vi "calcVectorField.vi"(7 "m":u32, 8 "error (in)":errorcluster, 10 "Boundary Points (1D)":cluster{"x":dbl, "y":dbl}[](array[cluster]), 11 "Interior Points (1D)":cluster{"x":dbl, "y":dbl}[](array[cluster])) -> (0 "error (out)":errorcluster, 1 "divergence(Fx, Fy)":dbl[][](array[numeric]), 2 "Y Vector Component":dbl[][](array[numeric]), 3 "X Vector Component":dbl[][](array[numeric]), 4 "curl(Fx, Fy)":dbl[][](array[numeric]))   [LabVIEW 2015]
uses:
  <vilib>/Analysis/baseanly.llb/Unit Vector (DBL).vi
  <vilib>/imath/engines/lvmath2/RunTimeEngine/Managers/WorkSpace/UID Generator.vi
  <vilib>/imath/engines/lvmath2/RunTimeEngine/BuiltInFunctions/divergence/NIMS_divergence(M,M).vi
  <vilib>/imath/engines/lvmath2/RunTimeEngine/RunTimeType/NIMS_RunTimeType_From StrictType (excl LVString).vi
  <instcachedir>/0/NIMS_RunTimeType_From StrictType (excl LVString)_EB1C38A9BC5048DA9ABDA8F781E54D21.lvgen/NIMS_RunTimeType_From StrictType (excl LVString)_EB1C38A9BC5048DA9ABDA8F781E54D21_000.vi
  <vilib>/imath/engines/lvmath2/RunTimeEngine/ErrorHandling/NIMS_Error From Error Code.vi
  <vilib>/imath/engines/lvmath2/RunTimeEngine/LocalVariableDefStatement/MC_LocalVariableDefStatement_Display.vi
  <vilib>/imath/engines/lvmath2/RunTimeEngine/BuiltInFunctions/curl/NIMS_[2o]_curl(M,M).vi
  <vilib>/imath/engines/lvmath2/RunTimeEngine/Managers/SymbolTable/Clear UID.vi
  <vilib>/imath/engines/lvmath2/RunTimeEngine/NodeEndStatement/NIMS_NodeEndStatement_Output.vi
  <instcachedir>/0/NIMS_NodeEndStatement_Output_53EC0D466D134D7ABD903AC30B43404B.lvgen/NIMS_NodeEndStatement_Output_53EC0D466D134D7ABD903AC30B43404B_002.vi
  <vilib>/imath/engines/lvmath2/RunTimeEngine/ErrorHandling/NIMS_Finalize Error.vi
  <vilib>/express/express arith-compare/Formula/XNode/ExpressFormulaBlockNode.xnode
  <vilib>/Analysis/NI_AALBase.lvlib
  <vilib>/imath/engines/lvmath2/RunTimeEngine/Managers/SymbolTable/NIMS_WorkSpace.lvlib
panel:
  out "-m":dbl
  out "m+2":dbl
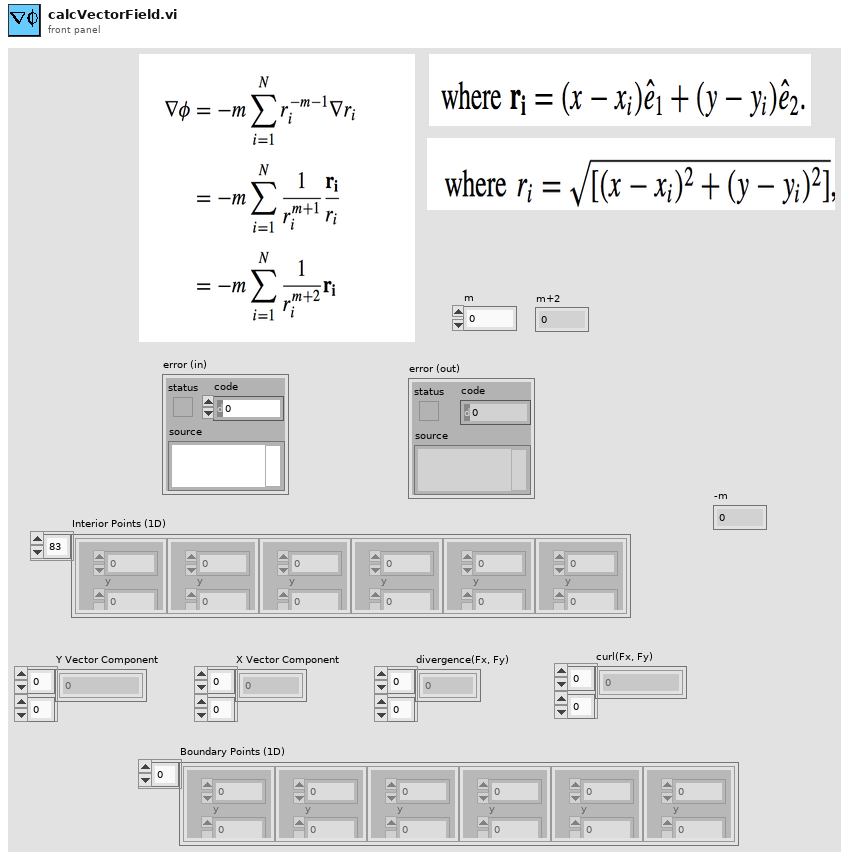
[diagram p1: front panel]
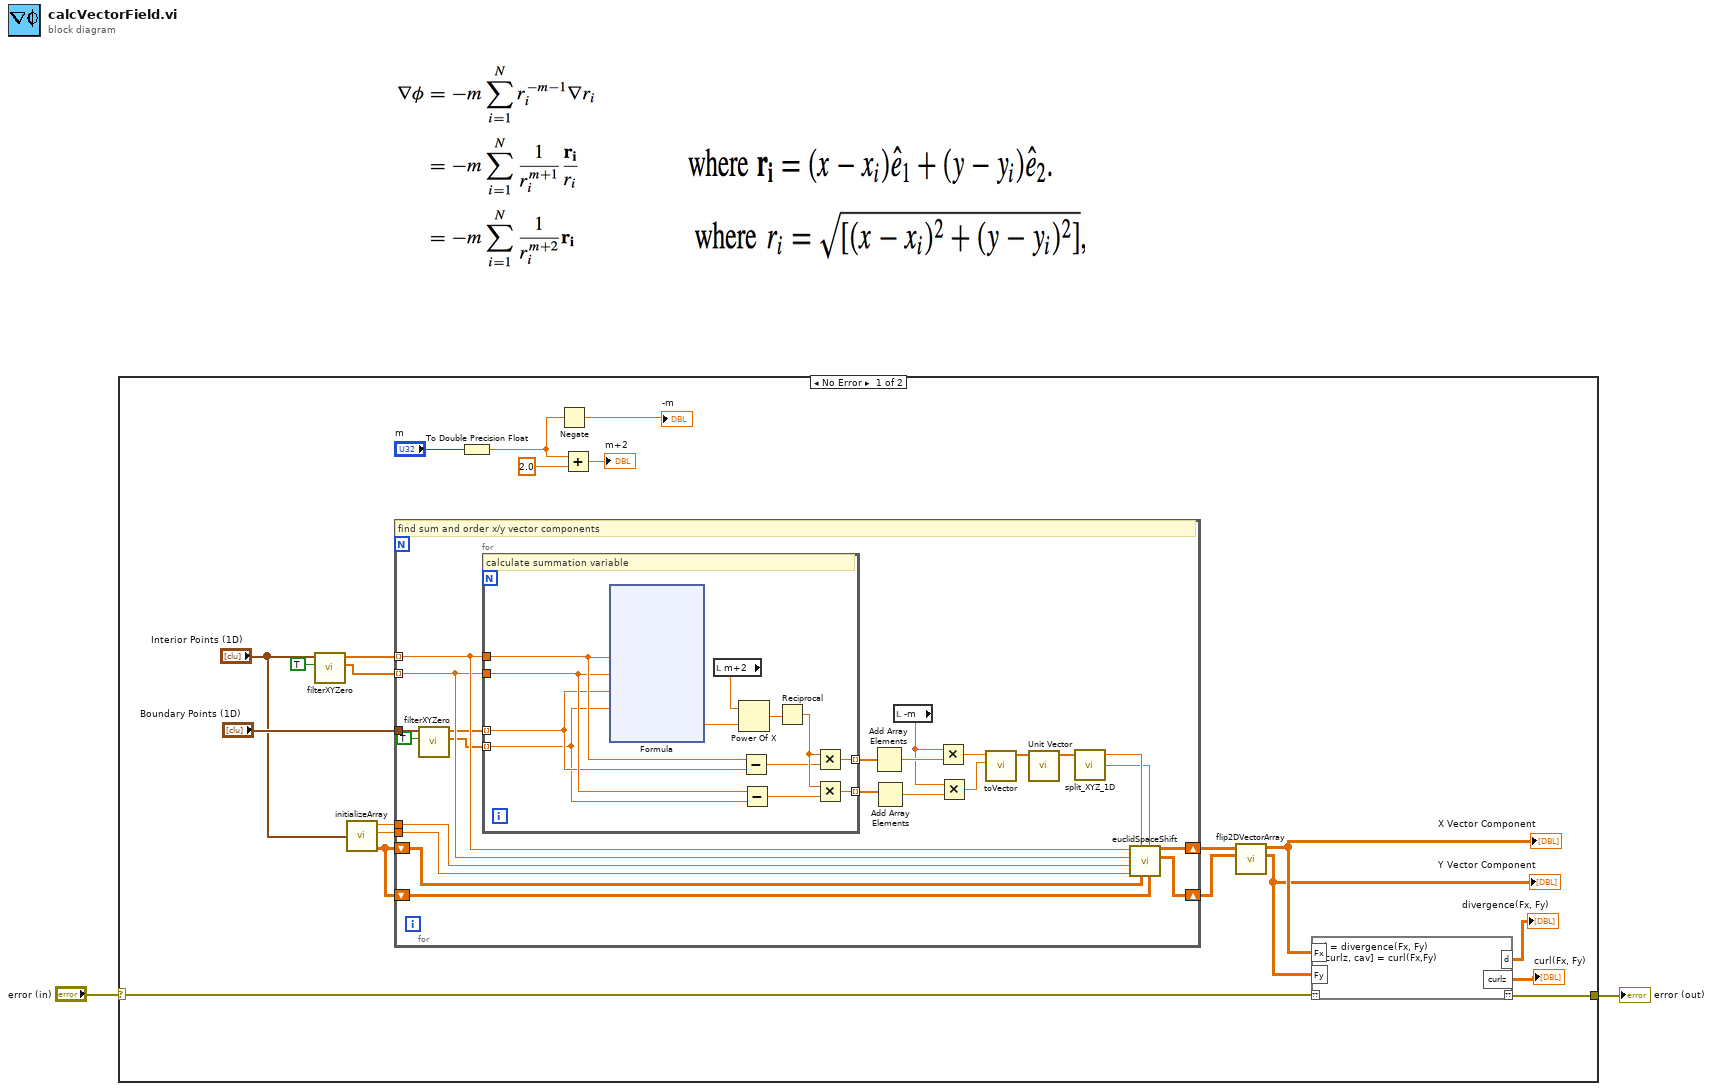
[diagram p0: block diagram]
diagram:
  n1 = case shown="No Error" "error (in)" {
    selector: "error (in)" -> [w5 w152]
    tunnel: [w4 w152] -> w1
    frame No Error {
      n2 = call "filterXYZero.vi"("Filter Zero?"=TRUE, "Points"="Interior Points (1D)") -> ("Y"=w12:dbl[], "X"=w13:dbl[])  [unwired: 7 in, 1 out]
      n3 = call "initializeArray.vi"("Interior Points (1D)"="Interior Points (1D)") -> ("XMin"=w22:dbl, "YMin"=w21:dbl, "initialized array"=w8:dbl[][])  [unwired: 1 in]
      n4 = for {
        shift-right: [w121] -> w10
        shift-left: w8 -> [w117]
        shift-right: [w120] -> w9
        shift-left: w8 -> [w116]
        tunnel: w22 -> [w119]
        tunnel: w21 -> [w118]
        tunnel: "Boundary Points (1D)" -> [w110]
        tunnel: w13 -> [w112] mode=indexing
        tunnel: w12 -> [w111] mode=indexing
        # "find sum and order x/y vector components"
        n5 = call "filterXYZero.vi"("Filter Zero?"=TRUE, "Points"=w110) -> ("Y"=w108:dbl[], "X"=w109:dbl[])  [unwired: 7 in, 1 out]
        n6 = for {
          tunnel: w112 -> [w134]
          tunnel: w111 -> [w133]
          tunnel: [w132] -> w123 mode=indexing
          tunnel: [w131] -> w122 mode=indexing
          tunnel: w109 -> [w127] mode=indexing
          tunnel: w108 -> [w126] mode=indexing
          # "calculate summation variable"
          n7 = xnode "Formula"("x"=w134, "y"=w133, "xB"=w127, "yB"=w126) -> ("Result"=w135:dbl)  [unwired: 1 in, 1 out]
          n8 = local read "m+2"() -> (w128:dbl)
          n9 = Power Of X(1:w135, 2:w128) -> (0:w137:dbl)
          n10 = Subtract(x=w134, y=w127) -> (x-y=w130:dbl)
          n11 = Subtract(x=w133, y=w126) -> (x-y=w129:dbl)
          n12 = Reciprocal(x=w137) -> (1/x=w136:dbl)
          n13 = Multiply(x=w136, y=w130) -> (x*y=w132:dbl)
          n14 = Multiply(x=w136, y=w129) -> (x*y=w131:dbl)
        }
        n15 = Add Array Elements(numeric array=w123) -> (sum=w124:dbl)
        n16 = Add Array Elements(numeric array=w122) -> (sum=w125:dbl)
        n17 = local read "-m"() -> (w113:dbl)
        n18 = Multiply(x=w113, y=w124) -> (x*y=w105:dbl)
        n19 = Multiply(x=w113, y=w125) -> (x*y=w106:dbl)
        n20 = call "toVector.vi"("Y Component"=w106, "X Component"=w105) -> ("Vector <x,y>"=w115:dbl[])  [unwired: 9 in]
        n21 = call-poly <vilib>:"Unit Vector.vi"("Input Vector"=w115) -> ("Unit Vector"=w114:dbl[])  [unwired: 8 in, 2 out]
        n22 = call "split_XYZ_1D.vi"("Point"=w114) -> ("X"=w104:dbl, "Y"=w103:dbl)  [unwired: 1 out]
        n23 = call "euclidSpaceShift.vi"("Y Vector Initialized Array"=w116, "Y Vector Component"=w103, "X Vector Initialized Array"=w117, "X Vector Component"=w104, "YMin"=w118, "XMin"=w119, "Y(i)"=w111, "X(i)"=w112) -> ("Y Vector Component Array"=w120:dbl[][], "X Vector Component Array"=w121:dbl[][])  [unwired: 2 in]
      }
      n24 = To Double Precision Float(number="m") -> (double precision float=w17:dbl)
      n25 = Negate(x=w17) -> (-x=→"-m":dbl)
      n26 = Add(x=w17, y=2.0) -> (x+y=→"m+2":dbl)
      n27 = call "flip2DVectorArray.vi"("Y Vector Component Array"=w9, "X Vector Component Array"=w10) -> ("Y Vector Component"=w6:dbl[][], "X Vector Component"=w7:dbl[][])  [unwired: 8 in]
      "X Vector Component" <- w7
      "Y Vector Component" <- w6
      n28 = mathscript code="d = divergence(Fx, Fy)\n[curlz, cav] = curl(Fx,Fy)"("??"=w5, "Fx"=w7, "Fy"=w6) -> ("??"=w4:errorcluster, "d"=→"divergence(Fx, Fy)":dbl[][], "curlz"=→"curl(Fx, Fy)":dbl[][])
    }
    frame Error {
    }
  }
  "error (out)" <- w1
